vi "parse packet.vi"(8 "error in (no error)":errorcluster, 11 "data passing":T1) -> (0 "error out":errorcluster, 1 "parameters":string, 2 "opcode":string, 3 "data passing out":T1)   [LabVIEW 2016]
uses:
  data.ctl
  device/device.ctl
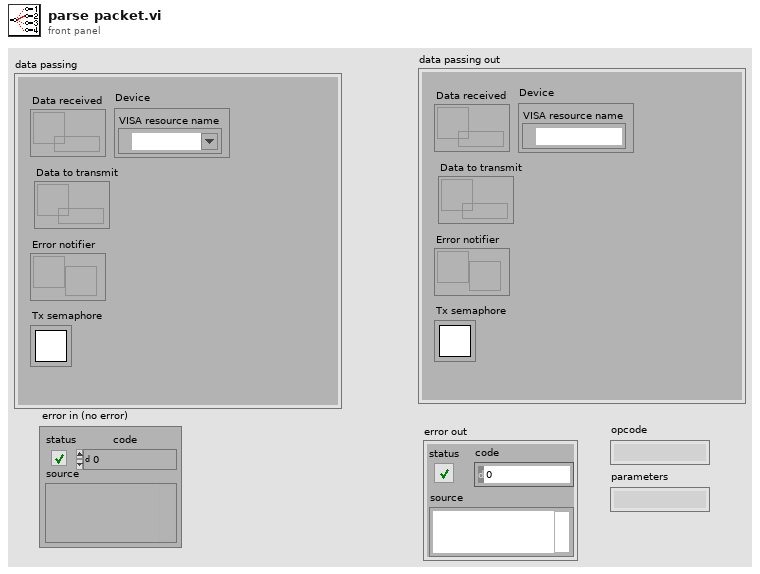
[diagram p1: front panel]
types:
  T1 = typedef "data.ctl" = cluster{"Data received":refnum<queue>, "Data to transmit":refnum<queue>, "Error notifier":refnum<notifier>, "Tx semaphore":T2, "Device":T3}
  T2 = typedef "Semaphore RefNum" = refnum<k1>
  T3 = typedef "device.ctl" = cluster{"VISA resource name":refnum<visa-resource-name>}
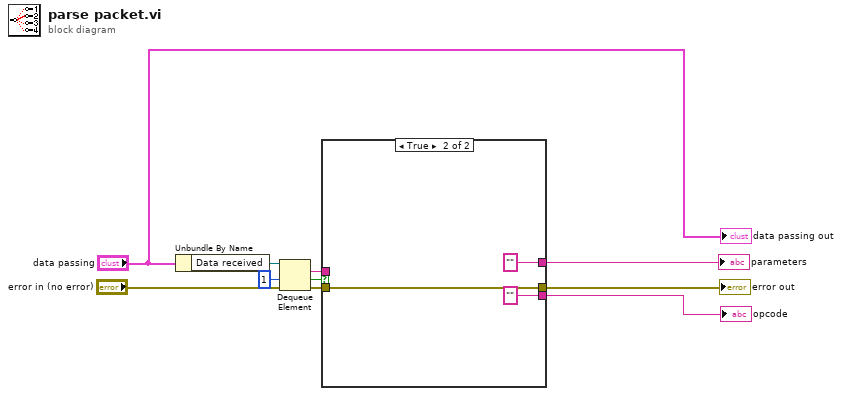
[diagram p0: block diagram]
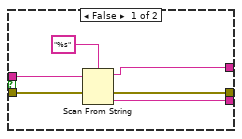
[diagram p2: hidden frame]
diagram:
  n1 = Unbundle By Name("data passing") -> ("Data received"=w10:refnum<queue>)
  n2 = Dequeue Element(queue=w10, timeout in ms (-1)=1, error in (no error)="error in (no error)") -> (element=w8:string, timed out?=w6:bool, error out=w7:errorcluster)  [unwired: 1 out]
  n3 = case shown="True" w6 {
    tunnel: w8 -> [w16 _]
    tunnel: w7 -> [w15 w19]
    tunnel: [w11 w19] -> w3
    tunnel: [w13 ""] -> w2
    tunnel: [w12 ""] -> w1
    frame False {
      n4 = Scan From String(format string="%s", input string=w16, error in=w15) -> (remaining string=w13:string, error out=w11:errorcluster, output 1=w12:string)  [unwired: 2 in, 1 out]
    }
    frame True {
    }
  }
  "error out" <- w3
  "opcode" <- w1
  "parameters" <- w2
  "data passing out" <- "data passing"
